vi "Main.vi"() -> ()   [LabVIEW 2017]
doc: "This template is for the Queued Message Handler design pattern.\n\nThe Event Handling Loop generates messages based on user interface actions.\n\nThe Message Handling Loop processes messages generated by the Event Handling Loop, or by other messages. The messages are string values, so new messages can be added easily to the Message Cases case structure in the Message Handling Loop. Each message cluster can also provide an optional value for Message Data, which is a variant that can be converted to whatever message-specific data is required."
uses:
  Position Slider.ctl
  Wash Step Controls.ctl
  Entry Display Data.ctl
  Wash Step Indicators.ctl
  support/Message Queue/Enqueue Message (Single).vi
  <vilib>/Utility/error.llb/Error Cluster From Error Code.vi
  <vilib>/ErrorRing/Error Ring.xnode
  support/Message Queue/Message Queue.lvlib
  support/User Event - Stop/User Event - Stop.lvlib
panel:
  in  "Wash step selection buttons":T1
  in  "Car Position Slider":T2 scale=0.0..4.0
  in  "Start":bool
  in  "Do Something <Replace Me>":bool
  in  "Exit":bool
  # "These controls have associated \"Value Changed\" events configured in the Event Structure on the diagram.\n\nReplace them (and reconfigure the Event Structure) with the controls you need for your application."
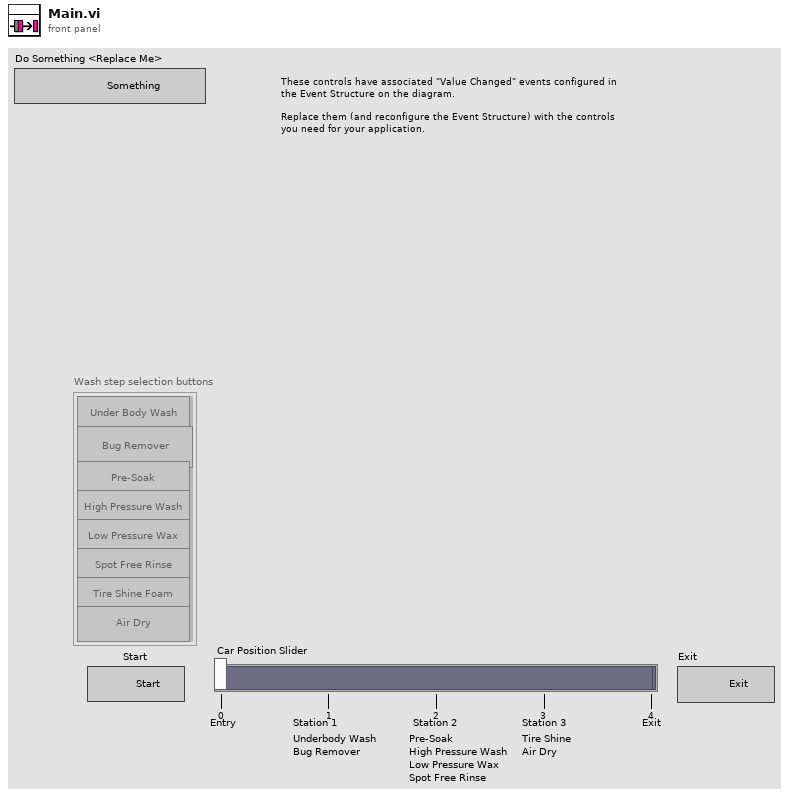
[diagram p1: front panel]
types:
  T1 = typedef "Wash Step Controls.ctl" = cluster{"Under Body Wash":bool, "Bug Remover":bool, "Pre-Soak":bool, "High Pressure Wash":bool, "Low Pressure Wax":bool, "Spot Free Rinse":bool, "Tire Shine Foam":bool, "Air Dry":bool}
  T2 = typedef "Position Slider.ctl" = i32
  T3 = typedef "Entry Display Data.ctl" = cluster{"Wash Entry Display":bool, "Car Position Slider":T2, "Wash Display Indicators":T4, "Vehicle Postion":bool}
  T4 = typedef "Wash Step Indicators.ctl" = cluster{"Under Body Wash":bool, "Bug Remover":bool, "Pre-soak":bool, " High Pressure Wash":bool, "Low Pressure  Wax":bool, "Spot Free Rinse":bool, " Tire Shine Foam":bool, " Air Dry":bool}
  T5 = typedef "Message Queue.lvlib/All Message Queues.ctl" = cluster{"MHL":refnum<queue>, "Controller":refnum<queue>, "Display":refnum<queue>}
  T6 = enum8{"Enabled", "Disabled", "Disabled and Grayed Out"}
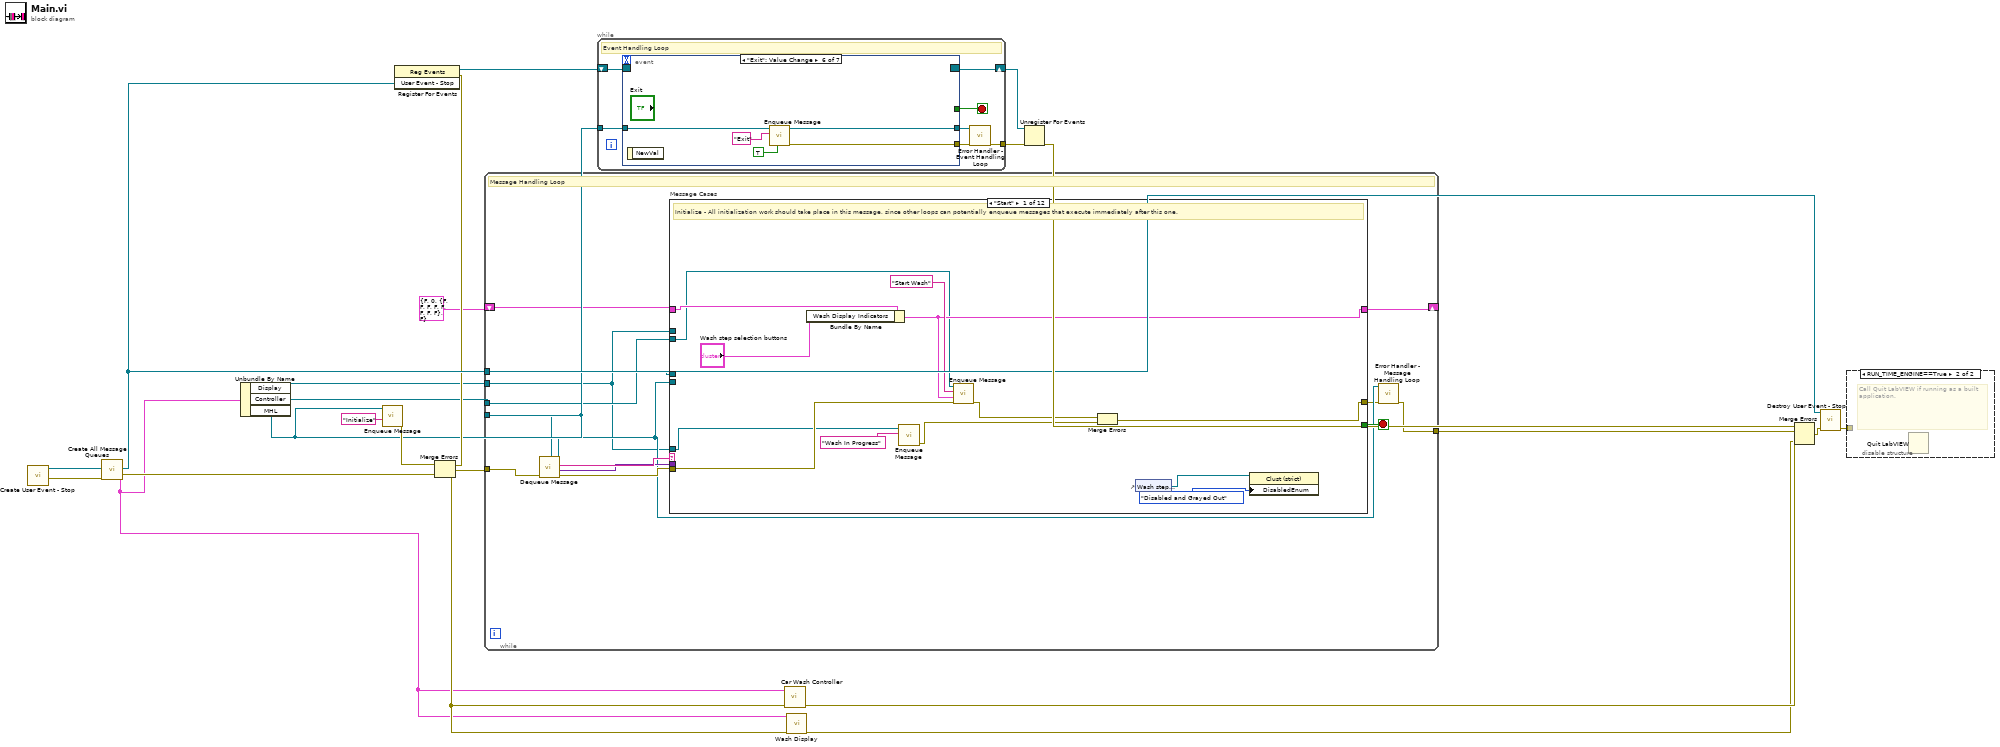
[diagram p0: block diagram]
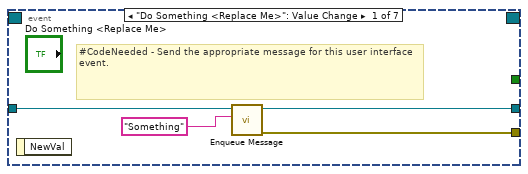
[diagram p3: hidden frame]
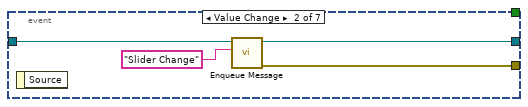
[diagram p4: hidden frame]
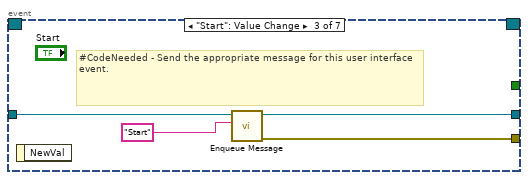
[diagram p5: hidden frame]
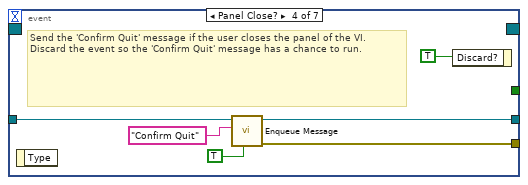
[diagram p6: hidden frame]
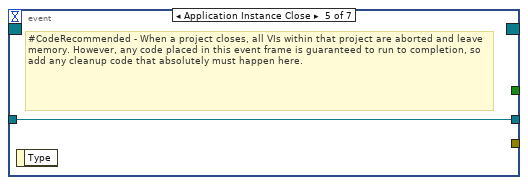
[diagram p7: hidden frame]
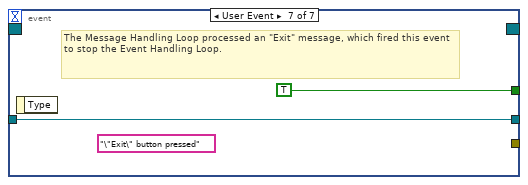
[diagram p8: hidden frame]
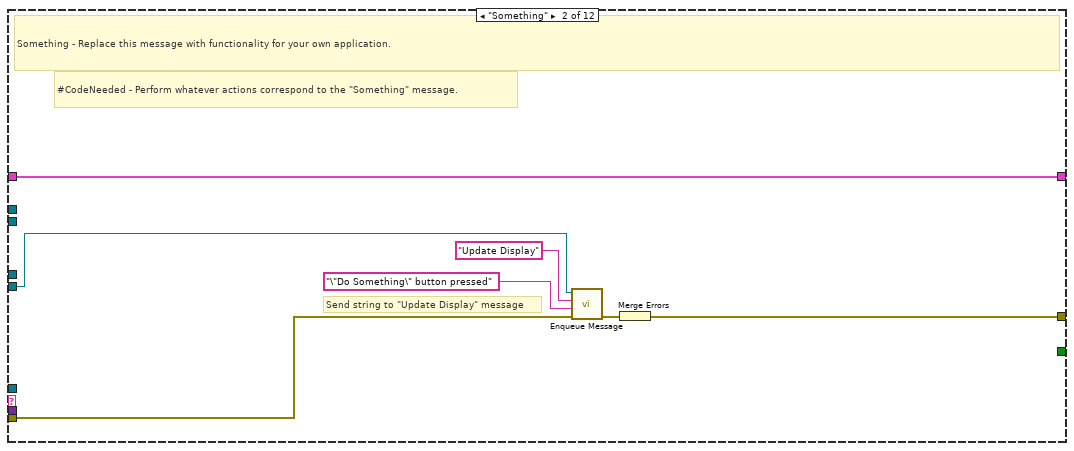
[diagram p9: hidden frame]
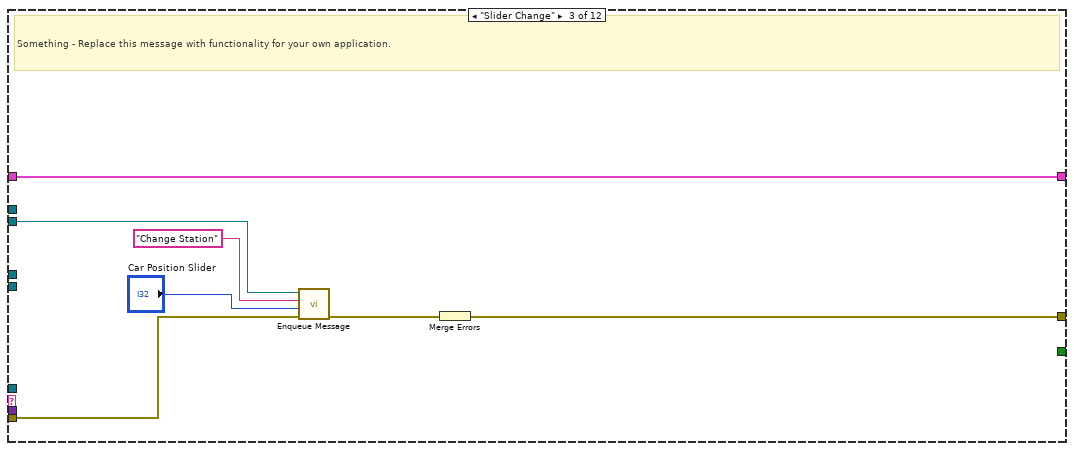
[diagram p10: hidden frame]
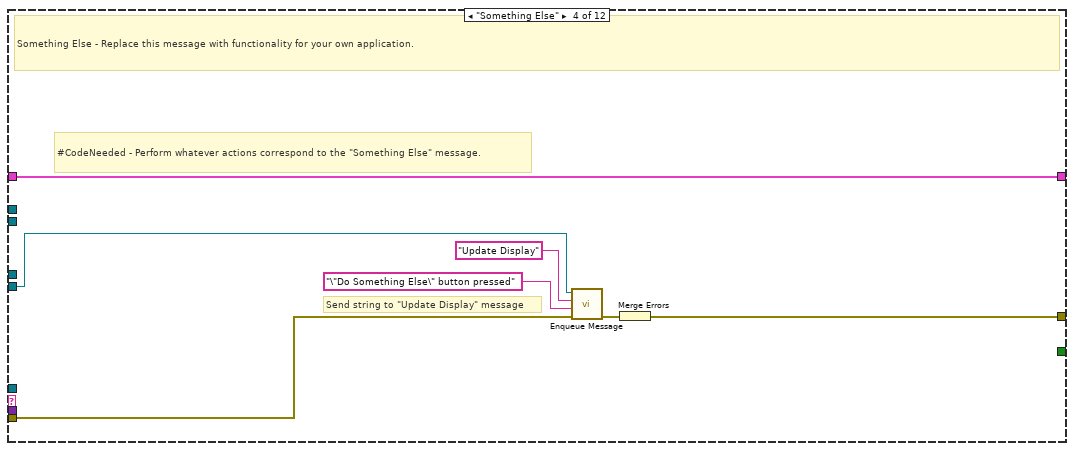
[diagram p11: hidden frame]
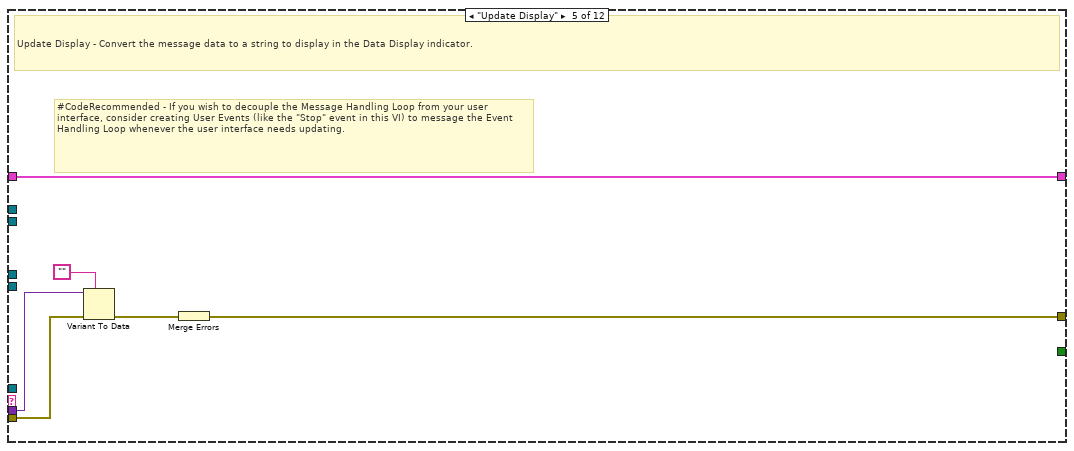
[diagram p12: hidden frame]
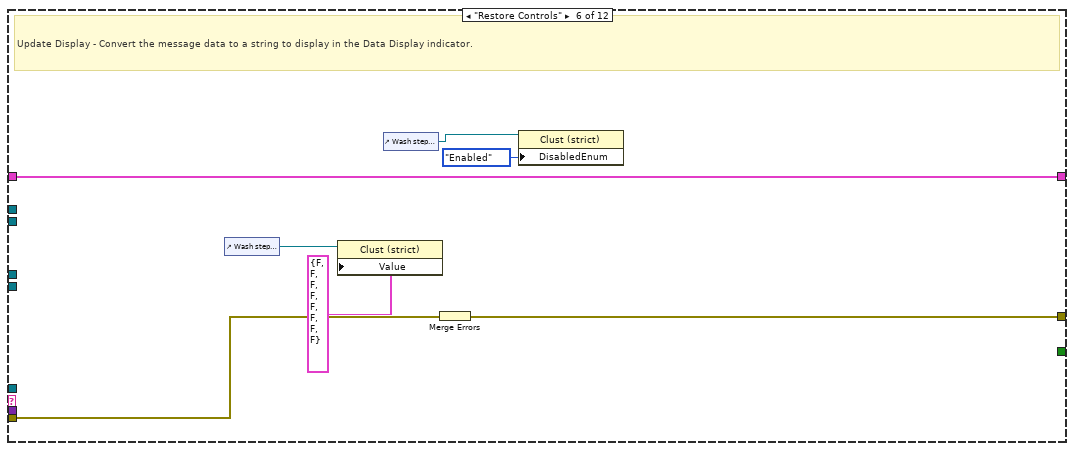
[diagram p13: hidden frame]
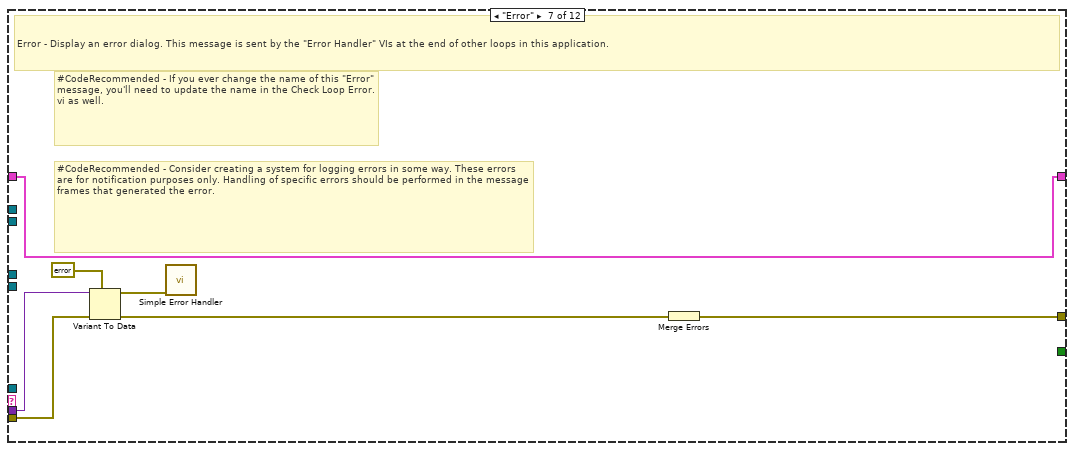
[diagram p14: hidden frame]
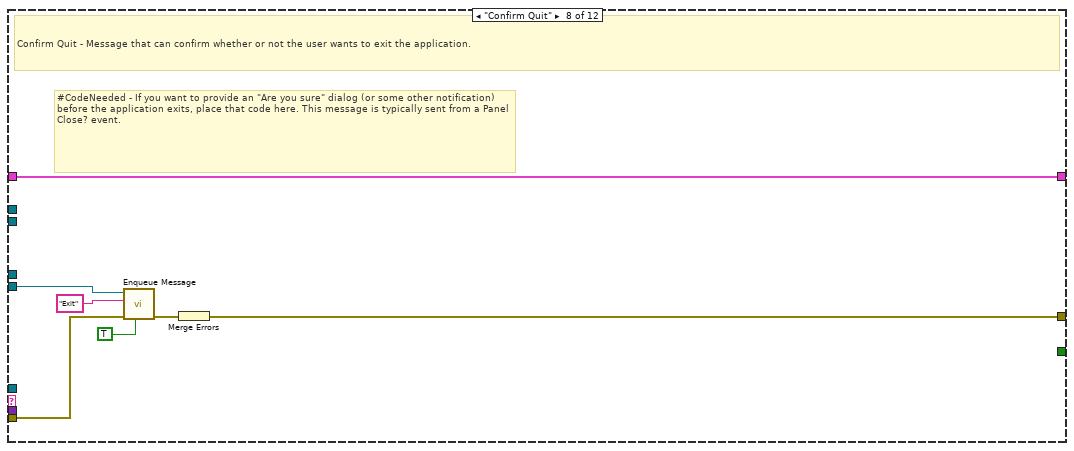
[diagram p15: hidden frame]
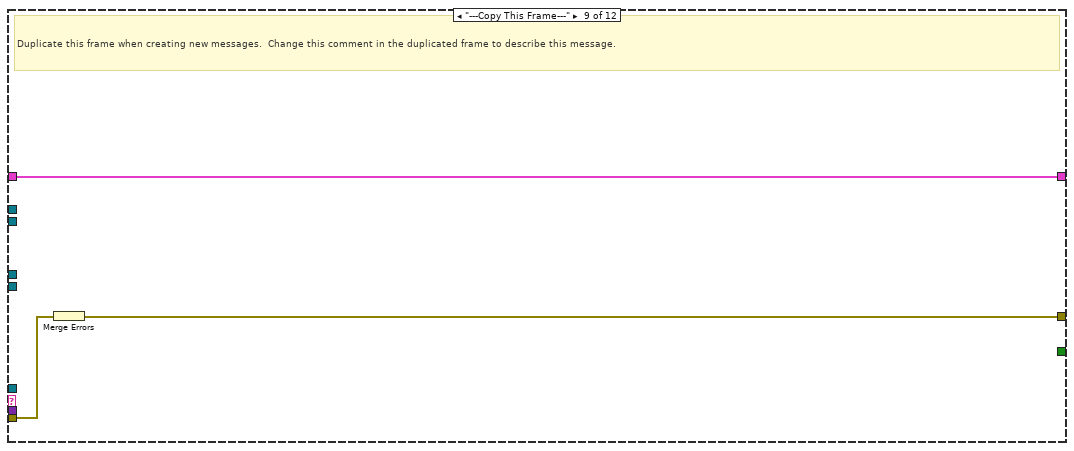
[diagram p16: hidden frame]
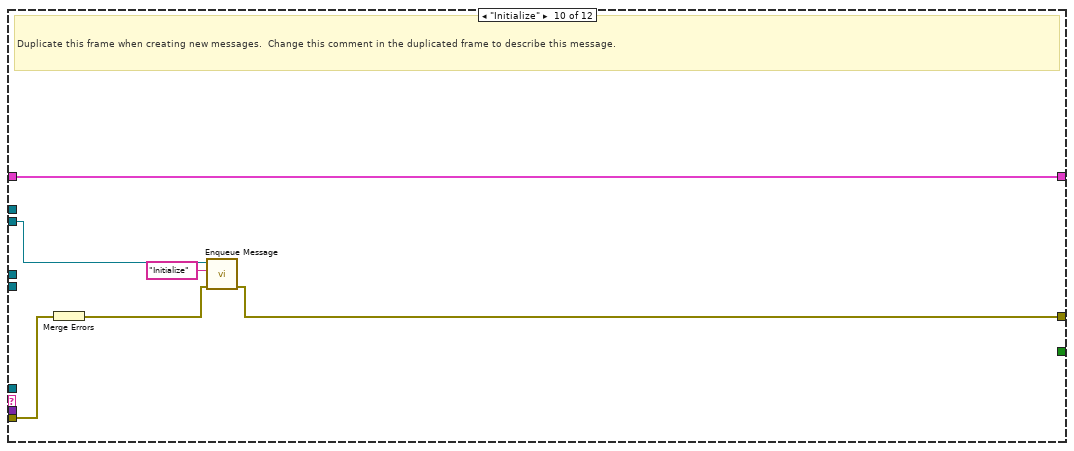
[diagram p17: hidden frame]
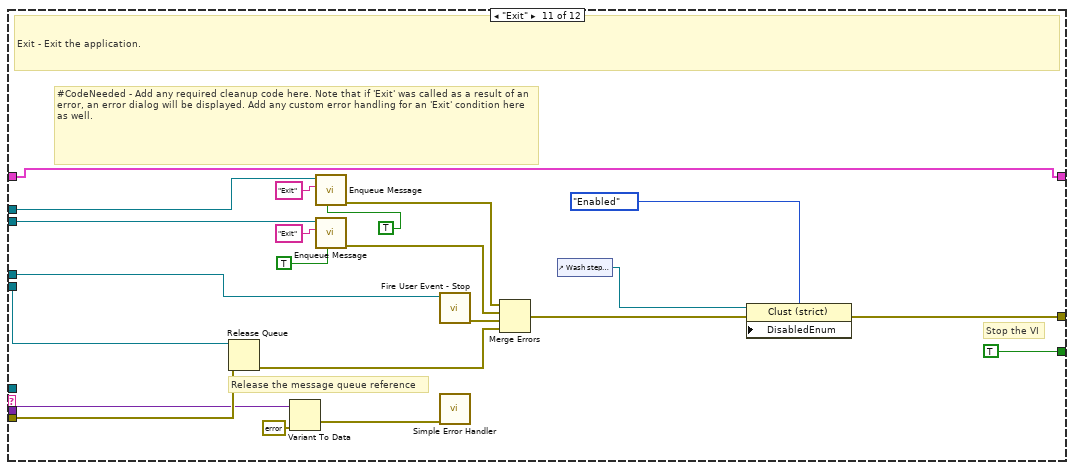
[diagram p18: hidden frame]
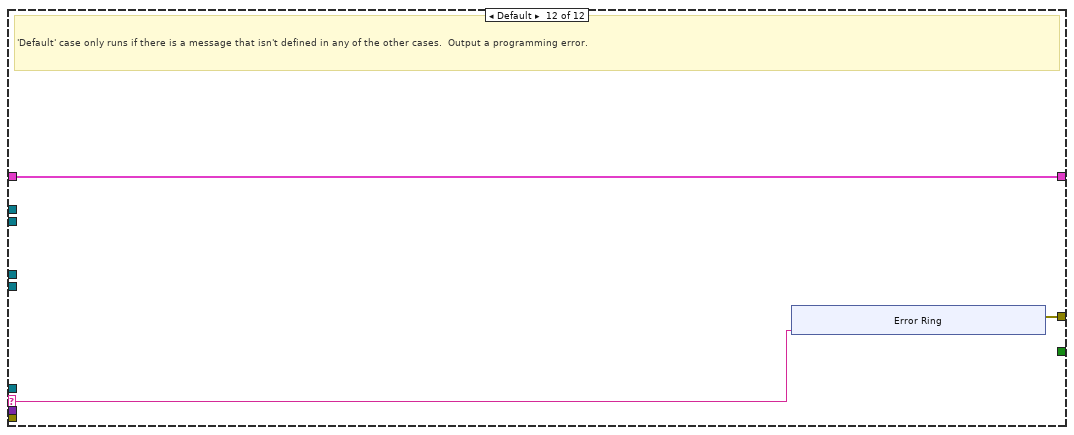
[diagram p19: hidden frame]
diagram:
  n1 = call "Create User Event - Stop.vi"() -> ("error out"=w20:errorcluster, "User Event - Stop"=w13:refnum<user-event>)  [unwired: 10 in]
  n2 = call "Create All Message Queues.vi"("error in (no error)"=w20) -> ("error out"=w7:errorcluster, "Message Queues out"=w1:T5)  [unwired: 9 in]
  n3 = Unbundle By Name(w1) -> ("Display"=w8:refnum<queue>, "Controller"=w6:refnum<queue>, "MHL"=w3:refnum<queue>)
  n4 = call-poly "Enqueue Message.vi"("Message"="Initialize", "Message Queue"=w3) -> ("error out"=w4:errorcluster)  [unwired: 8 in, 1 out]
  n5 = register-events(w13) -> (reference out=w14:refnum<event-registration>, error out=w12:errorcluster)  [unwired: 2 in]
  n6 = Merge Errors(w4, w12, w7) -> (w2:errorcluster)
  n7 = while {
    tunnel: w3 -> [w27]
    shift-right: [w34] -> _
    shift-left: T3 {"Wash Entry Display"=FALSE, "Car Position Slider"=0, "Wash Display Indicators"={"Under Body Wash"=FALSE, "Bug Remover"=FALSE, "Pre-soak"=FALSE, " High Pressure Wash"=FALSE, "Low Pressure  Wax"=FALSE, "Spot Free Rinse"=FALSE, " Tire Shine Foam"=FALSE, " Air Dry"=FALSE}, "Vehicle Postion"=FALSE} ("Cluster") -> [w35]
    tunnel: w13 -> [w32]
    tunnel: w2 -> [w31]
    tunnel: [w25] -> w21
    tunnel: w6 -> [w23]
    tunnel: w8 -> [w22]
    stop <- w33 stop-if-true
    # "Message Handling Loop"
    n8 = call "Dequeue Message.vi"("error in (no error)"=w31, "Message Queue"=w27) -> ("error out"=w30:errorcluster, "Message Data"=w28:variant, "Message"=w29:string, "dup Message Queue"=w26:refnum<queue>)  [unwired: 6 in]
    n9 = case "Message Cases" shown="\"Start\"" w29 {
      selector: w29 -> [_ _ _ _ _ _ _ _ _ _ _ w128]
      tunnel: w26 -> [_ w51 _ w65 _ _ _ w92 _ _ w127 _]
      tunnel: w30 -> [w48 w53 w61 w67 w73 w80 w89 w96 w99 w105 w121 _]
      tunnel: [w37 w54 w62 w68 w74 w81 w83 w94 w97 w100 w107 w129] -> w24
      tunnel: w35 -> [w46 w55 w58 w69 w75 w82 w88 w95 w98 w104 w126 w130]
      tunnel: [w45 w55 w58 w69 w75 w82 w88 w95 w98 w104 w126 w130] -> w34
      tunnel: [_ _ _ _ _ _ _ _ _ _ TRUE _] -> w33
      tunnel: w28 -> [_ _ _ _ w72 _ w87 _ _ _ w119 _]
      tunnel: w32 -> [_ _ _ _ _ _ _ _ _ _ w123 _]
      tunnel: w23 -> [w44 _ w57 _ _ _ _ _ _ w103 w118 _]
      tunnel: w22 -> [_ _ _ _ _ _ _ _ _ _ w114 _]
      tunnel: w22 -> [w40 _ _ _ _ _ _ _ _ _ _ _]
      frame "Start" {
        # "Initialize - All initialization work should take place in this message, since other loops can potentially enqueue messages that execute immediately after this one."
        n10 = Bundle By Name(cluster=w46, "Wash Display Indicators"="Wash step selection buttons") -> (w45:T3)
        n11 = call-poly "Enqueue Message.vi"("Message"="Wash In Progress", "Message Queue"=w40) -> ("error out"=w38:errorcluster)  [unwired: 8 in, 1 out]
        n12 = call-poly "Enqueue Message.vi"("error in (no error)"=w48, "Message Data"=w45, "Message"="Start Wash", "Message Queue"=w44) -> ("error out"=w39:errorcluster)  [unwired: 6 in, 1 out]
        n13 = Merge Errors(w39, w38) -> (w37:errorcluster)
        n14 = control-ref of="Wash step selection buttons"() -> (w42:refnum<vi>)
        n15 = property class="Clust (strict)"(reference=w42, "DisabledEnum"=T6."Disabled and Grayed Out" ("Disabled")) -> ()  [unwired: 1 in, 2 out]
      }
      frame "Something" {
        # "Send string to \"Update Display\" message"
        # "#CodeNeeded - Perform whatever actions correspond to the \"Something\" message."
        # "Something - Replace this message with functionality for your own application."
        n16 = call-poly "Enqueue Message.vi"("error in (no error)"=w53, "Message Data"="\"Do Something\" button pressed" ("\"Do Something\" button pressed"), "Message"="Update Display", "Message Queue"=w51) -> ("error out"=w52:errorcluster)  [unwired: 6 in, 1 out]
        n17 = Merge Errors(w52) -> (w54:errorcluster)
      }
      frame "Slider Change" {
        # "Something - Replace this message with functionality for your own application."
        n18 = call-poly "Enqueue Message.vi"("error in (no error)"=w61, "Message Data"="Car Position Slider", "Message"="Change Station", "Message Queue"=w57) -> ("error out"=w60:errorcluster)  [unwired: 6 in, 1 out]
        n19 = Merge Errors(w60) -> (w62:errorcluster)
      }
      frame "Something Else" {
        # "Send string to \"Update Display\" message"
        # "#CodeNeeded - Perform whatever actions correspond to the \"Something Else\" message."
        # "Something Else - Replace this message with functionality for your own application."
        n20 = call-poly "Enqueue Message.vi"("error in (no error)"=w67, "Message Data"="\"Do Something Else\" button pressed" ("\"Do Something Else\" button pressed"), "Message"="Update Display", "Message Queue"=w65) -> ("error out"=w66:errorcluster)  [unwired: 6 in, 1 out]
        n21 = Merge Errors(w66) -> (w68:errorcluster)
      }
      frame "Update Display" {
        # "#CodeRecommended - If you wish to decouple the Message Handling Loop from your user interface, consider creating User Events (like the \"Stop\" event in this VI) to message the Event Handling Loop whenever the user interface needs updating."
        # "Update Display - Convert the message data to a string to display in the Data Display indicator."
        n22 = Variant To Data(error in=w73, type="", Variant=w72) -> (error out=w70:errorcluster)  [unwired: 1 out]
        n23 = Merge Errors(w70) -> (w74:errorcluster)
      }
      frame "Restore Controls" {
        # "Update Display - Convert the message data to a string to display in the Data Display indicator."
        n24 = control-ref of="Wash step selection buttons"() -> (w79:refnum<vi>)
        n25 = property class="Clust (strict)"(reference=w79, "Value"=T1 {"Under Body Wash"=FALSE, "Bug Remover"=FALSE, "Pre-Soak"=FALSE, "High Pressure Wash"=FALSE, "Low Pressure Wax"=FALSE, "Spot Free Rinse"=FALSE, "Tire Shine Foam"=FALSE, "Air Dry"=FALSE}) -> ()  [unwired: 1 in, 2 out]
        n26 = control-ref of="Wash step selection buttons"() -> (w77:refnum<vi>)
        n27 = Merge Errors(w80) -> (w81:errorcluster)
        n28 = property class="Clust (strict)"(reference=w77, "DisabledEnum"=T6."Enabled" ("Disabled")) -> ()  [unwired: 1 in, 2 out]
      }
      frame "Error" {
        # "#CodeRecommended - If you ever change the name of this \"Error\" message, you'll need to update the name in the Check Loop Error.vi as well."
        # "#CodeRecommended - Consider creating a system for logging errors in some way. These errors are for notification purposes only. Handling of specific errors should be performed in the message frames that generated the error."
        # "Error - Display an error dialog. This message is sent by the \"Error Handler\" VIs at the end of other loops in this application."
        n29 = Variant To Data(error in=w89, type=errorcluster {"status"=FALSE, "code"=0, "source"=""} ("error constant"), Variant=w87) -> (data=w85:errorcluster, error out=w84:errorcluster)
        n30 = call <vilib>:"Simple Error Handler.vi"("error in (no error)"=w85) -> ()  [unwired: 4 in, 5 out]
        n31 = Merge Errors(w84) -> (w83:errorcluster)
      }
      frame "Confirm Quit" {
        # "#CodeNeeded - If you want to provide an \"Are you sure\" dialog (or some other notification) before the application exits, place that code here. This message is typically sent from a Panel Close? event."
        # "Confirm Quit - Message that can confirm whether or not the user wants to exit the application."
        n32 = call-poly "Enqueue Message.vi"("Priority Message? (F)"=TRUE, "error in (no error)"=w96, "Message"="Exit", "Message Queue"=w92) -> ("error out"=w93:errorcluster)  [unwired: 6 in, 1 out]
        n33 = Merge Errors(w93) -> (w94:errorcluster)
      }
      frame "---Copy This Frame---" {
        # "Duplicate this frame when creating new messages.  Change this comment in the duplicated frame to describe this message."
        n34 = Merge Errors(w99) -> (w97:errorcluster)
      }
      frame "Initialize" {
        # "Duplicate this frame when creating new messages.  Change this comment in the duplicated frame to describe this message."
        n35 = Merge Errors(w105) -> (w101:errorcluster)
        n36 = call-poly "Enqueue Message.vi"("error in (no error)"=w101, "Message"="Initialize", "Message Queue"=w103) -> ("error out"=w100:errorcluster)  [unwired: 7 in, 1 out]
      }
      frame "Exit" {
        # "Stop the VI"
        # "Release the message queue reference"
        # "#CodeNeeded - Add any required cleanup code here. Note that if 'Exit' was called as a result of an error, an error dialog will be displayed. Add any custom error handling for an 'Exit' condition here as well."
        # "Exit - Exit the application."
        n37 = Release Queue(queue=w127, error in (no error)=w121) -> (error out=w124:errorcluster)  [unwired: 1 in, 2 out]
        n38 = Variant To Data(error in=errorcluster {"status"=FALSE, "code"=0, "source"=""} ("error constant"), Variant=w119) -> (data=w120:errorcluster)  [unwired: 1 in, 1 out]
        n39 = call-poly "Enqueue Message.vi"("Priority Message? (F)"=TRUE, "Message"="Exit", "Message Queue"=w114) -> ("error out"=w112:errorcluster)  [unwired: 7 in, 1 out]
        n40 = call-poly "Enqueue Message.vi"("Priority Message? (F)"=TRUE, "Message"="Exit", "Message Queue"=w118) -> ("error out"=w115:errorcluster)  [unwired: 7 in, 1 out]
        n41 = call "Fire User Event - Stop.vi"("User Event - Stop"=w123) -> ("error out"=w122:errorcluster)  [unwired: 10 in]
        n42 = call <vilib>:"Simple Error Handler.vi"("error in (no error)"=w120) -> ()  [unwired: 4 in, 5 out]
        n43 = Merge Errors(w112, w115, w122, w124) -> (w108:errorcluster)
        n44 = control-ref of="Wash step selection buttons"() -> (w110:refnum<vi>)
        n45 = property class="Clust (strict)"(reference=w110, error in=w108, "DisabledEnum"=T6."Enabled" ("Disabled")) -> (error out=w107:errorcluster)  [unwired: 1 out]
      }
      frame Default {
        # "'Default' case only runs if there is a message that isn't defined in any of the other cases.  Output a programming error."
        n46 = xnode "Error Ring"("parameter 0"=w128) -> ("error out"=w129:errorcluster)
      }
    }
    n47 = call "Error Handler - Message Handling Loop.vi"("error in (no error)"=w24, "Message Queue"=w26) -> ("dup error in"=w25:errorcluster)  [unwired: 8 in, 1 out]
  }
  n48 = while {
    tunnel: w3 -> [w144]
    shift-right: [w142] -> w17
    shift-left: w14 -> [w143]
    tunnel: [w138] -> w15
    stop <- w140 stop-if-true
    # "Event Handling Loop"
    n49 = event shown="[5] \"Exit\": Value Change" {
      selector: w143 -> [_ _ _ _ _ _ _]
      dyn-events: [_ _ _ _ _ _ _] -> w142
      timeout: _ -> [_ _ _ _ _ _ _]
      tunnel: [_ _ _ _ _ _ TRUE ("Discard?")] -> w140
      tunnel: w144 -> [w148 w152 w156 w161 w163 w168 w170]
      tunnel: [w145 w149 w153 w160 _ w167 _] -> w141
      tunnel: [w147 w151 w155 w159 w163 w166 w170] -> w139
      event "Do Something <Replace Me>": Value Change {
        # "#CodeNeeded - Send the appropriate message for this user interface event."
        n50 = event-data() -> ()  [unwired: 1 in, 1 out]
        n51 = call-poly "Enqueue Message.vi"("Message"="Something", "Message Queue"=w148) -> ("error out"=w145:errorcluster, "dup Message Queue"=w147:refnum<queue>)  [unwired: 8 in]
      }
      event Value Change {
        n52 = event-data() -> ()  [unwired: 1 in, 1 out]
        n53 = call-poly "Enqueue Message.vi"("Message"="Slider Change", "Message Queue"=w152) -> ("error out"=w149:errorcluster, "dup Message Queue"=w151:refnum<queue>)  [unwired: 8 in]
      }
      event "Start": Value Change {
        # "#CodeNeeded - Send the appropriate message for this user interface event."
        n54 = event-data() -> ()  [unwired: 1 in, 1 out]
        n55 = call-poly "Enqueue Message.vi"("Message"="Start", "Message Queue"=w156) -> ("error out"=w153:errorcluster, "dup Message Queue"=w155:refnum<queue>)  [unwired: 8 in]
      }
      event Panel Close? {
        # "Send the 'Confirm Quit' message if the user closes the panel of the VI. Discard the event so the 'Confirm Quit' message has a chance to run."
        n56 = event-data() -> ()  [unwired: 1 in, 1 out]
        n57 = call-poly "Enqueue Message.vi"("Priority Message? (F)"=TRUE, "Message"="Confirm Quit", "Message Queue"=w161) -> ("error out"=w160:errorcluster, "dup Message Queue"=w159:refnum<queue>)  [unwired: 7 in]
        n58 = event-data("Discard?"=TRUE) -> ()  [unwired: 1 in, 1 out]
      }
      event Application Instance Close {
        # "#CodeRecommended - When a project closes, all VIs within that project are aborted and leave memory. However, any code placed in this event frame is guaranteed to run to completion, so add any cleanup code that absolutely must happen here."
        n59 = event-data() -> ()  [unwired: 1 in, 1 out]
      }
      event "Exit": Value Change {
        n60 = event-data() -> ()  [unwired: 1 in, 1 out]
        n61 = call-poly "Enqueue Message.vi"("Priority Message? (F)"=TRUE, "Message"="Exit", "Message Queue"=w168) -> ("error out"=w167:errorcluster, "dup Message Queue"=w166:refnum<queue>)  [unwired: 7 in]
      }
      event User Event {
        (unwired) "\"Exit\" button pressed" ("VI Stopped")
        # "The Message Handling Loop processed an \"Exit\" message, which fired this event to stop the Event Handling Loop."
        n62 = event-data() -> ()  [unwired: 1 in, 1 out]
      }
    }
    n63 = call "Error Handler - Event Handling Loop.vi"("error in (no error)"=w141, "Message Queue"=w139) -> ("dup error in"=w138:errorcluster)  [unwired: 8 in, 1 out]
  }
  n64 = call "Car Wash Controller.vi"("error in (no error)"=w2, "Message Queues"=w1) -> ("error out"=w11:errorcluster)  [unwired: 9 in]
  n65 = call "Wash Display.vi"("error in (no error)"=w2, "Message Queues"=w1) -> ("error out"=w9:errorcluster)  [unwired: 9 in]
  n66 = Unregister For Events(event registration refnum=w17, error in=w15) -> (error out=w18:errorcluster)
  n67 = Merge Errors(w18, w21, w11, w9) -> (w19:errorcluster)
  n68 = call "Destroy User Event - Stop.vi"("error in (no error)"=w19, "User Event - Stop"=w13) -> ("error out"=w16:errorcluster)  [unwired: 9 in]
  n69 = disable-structure shown="RUN_TIME_ENGINE==True" {
    disable-tunnel: w16 -> [_ _]
    frame condition #0 (active) {
    }
    frame condition #1 {
      # "Call Quit LabVIEW if running as a built application."
      n70 = Quit LabVIEW() -> ()  [unwired: 1 in]
    }
  }
